vi "1_5.vi"() -> ()   [LabVIEW 2010]
panel:
  out "Char":i16
  in  "stop":bool
  out "String":string
  in  "Numeric 2":dbl
  in  "Slide":dbl(slide) scale=0.0..10.0
  out "Numeric":i32
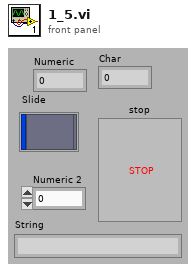
[diagram p1: front panel]
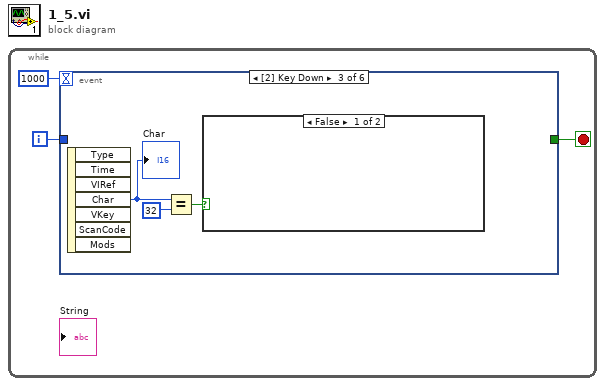
[diagram p0: block diagram]
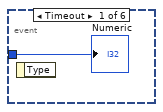
[diagram p2: hidden frame]
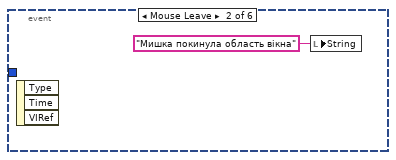
[diagram p3: hidden frame]
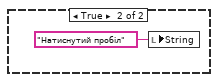
[diagram p4: hidden frame]
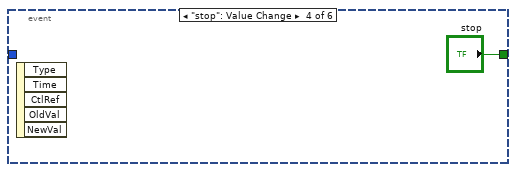
[diagram p5: hidden frame]
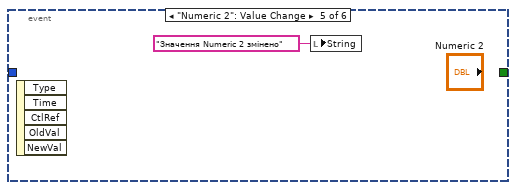
[diagram p6: hidden frame]
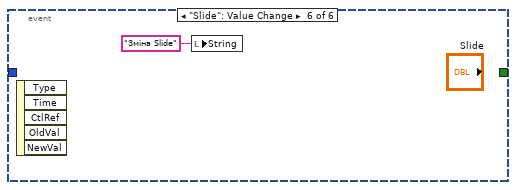
[diagram p7: hidden frame]
diagram:
  n1 = while {
    i -> [w2]
    stop <- w1 stop-if-true
    n2 = event shown="[2] Key Down" {
      selector: _ -> [_ _ _ _ _ _]
      dyn-events: _ -> [_ _ _ _ _ _]
      timeout: 1000 -> [_ _ _ _ _ _]
      tunnel: w2 -> [w4 _ _ _ _ _]
      tunnel: [_ _ _ "stop" _ _] -> w1
      event Timeout {
        n3 = event-data() -> ()  [unwired: 1 in, 1 out]
        "Numeric" <- w4
      }
      event Mouse Leave {
        n4 = event-data() -> ()  [unwired: 1 in, 3 out]
        n5 = local write "String"("Мишка покинула область вікна" ("String")) -> ()
      }
      event Key Down {
        n6 = event-data() -> ("Char"=w8:i16)  [unwired: 1 in, 6 out]
        "Char" <- w8
        n7 = Equal?(x=w8, y=i16 32) -> (x = y?=w6:bool)
        n8 = case shown="False" w6 {
          frame False {
          }
          frame True {
            n9 = local write "String"("Натиснутий пробіл" ("String")) -> ()
          }
        }
      }
      event "stop": Value Change {
        n10 = event-data() -> ()  [unwired: 1 in, 5 out]
      }
      event "Numeric 2": Value Change {
        n11 = event-data() -> ()  [unwired: 1 in, 5 out]
        n12 = local write "String"("Значення Numeric 2 змінено" ("String")) -> ()
      }
      event "Slide": Value Change {
        n13 = event-data() -> ()  [unwired: 1 in, 5 out]
        n14 = local write "String"("Зміна Slide" ("String")) -> ()
      }
    }
  }
